vi "setUp.vi"(8 "error in (no error)":errorcluster, 11 "reference in":refnum<class "Switch Consumer Test Case.lvclass">) -> (0 "error out":errorcluster, 3 "reference out":refnum<class "Switch Consumer Test Case.lvclass">)   [LabVIEW 2017, in "Switch Consumer Test Case.lvclass"]
doc: "setUp runs prior to the test method during test execution. Use this method to initialize any object data required by your tests."
uses:
  Switch Consumer Test Case.lvclass
  C:/Program Files (x86)/National Instruments/LabVIEW 2017/vi.lib/addons/_JKI Toolkits/VI Tester/TestCase.llb/TestCase.lvclass
  Support/Switch/Test Switch Consumer/Test Switch Consumer.lvclass
  C:/github/niveristand-custom-device-message-library/Source/Consumer/Abstract Consumer/Abstract Consumer.lvclass
  Support/Switch/Test Switch Init Parameters/Test Switch Init Parameters.lvclass
  C:/github/niveristand-custom-device-message-library/Source/Parameters/Abstract Init Parameters/Abstract Init Parameters.lvclass
  C:/github/niveristand-custom-device-message-library/Source/Switch/Abstract Switch Init Parameters/Abstract Switch Init Parameters.lvclass
  Message Queue/Message Queue/Message Queue.lvclass
  C:/github/niveristand-custom-device-message-library/Source/Message Queue/Abstract Message Queue/Abstract Message Queue.lvclass
  Parameters/Abstract Init Parameters/Abstract Init Parameters.lvclass
  Producer/Abstract Producer/Abstract Producer.lvclass
  Support/Message String Action.ctl
  Support/Message List Action.ctl
  Support/Switch/Test Switch Init Parameters/Test Switch Init Parameters.lvclass/Test Switch Init Parameters.ctl
  Switch Consumer Test Case.lvclass/Switch Consumer Test Case.ctl
  Support/Switch/Test Switch Init Parameters/Write Test Param.vi
  <vilib>/addons/_JKI Toolkits/VI Tester/TestCase.llb/TestCase.lvclass
  Consumer/Abstract Consumer/Abstract Consumer.lvclass
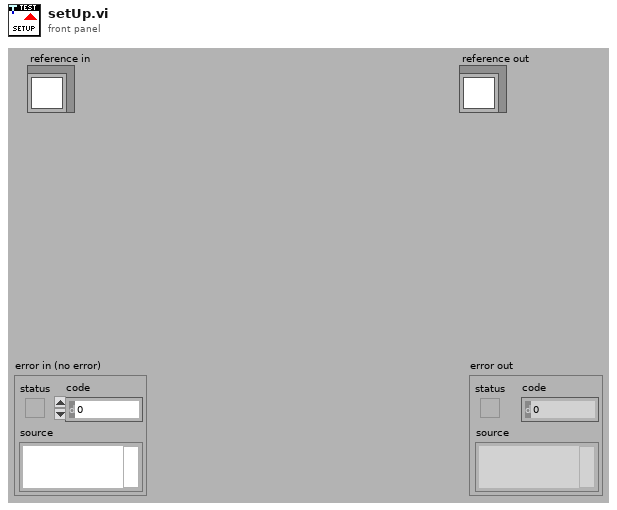
[diagram p1: front panel]
types:
  T1 = typedef "Message List Action.ctl" = enum16{"Get", "Add", "Reset"}
  T2 = typedef "Message String Action.ctl" = enum16{"Get String", "Set String", "Reset"}
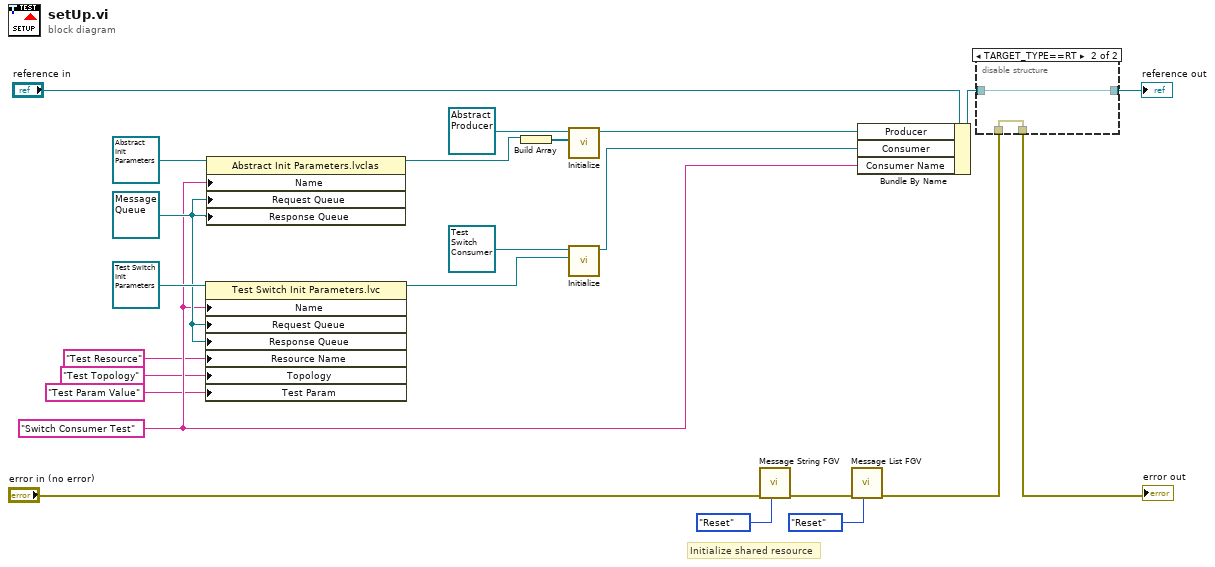
[diagram p0: block diagram]
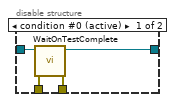
[diagram p2: hidden frame]
diagram:
  w9 = "Switch Consumer Test" ("Name")
  w17 = refnum<class "Message Queue.lvclass"> refnum ("Messaging.lvlib:Message Queue.lvlib:Message Queue.lvclass")
  # "Initialize shared resource"
  n1 = property class="Test Switch Init Parameters.lvc"(reference=refnum<class "Test Switch Init Parameters.lvclass"> refnum ("Test Switch Init Parameters.lvclass"), "Name"=w9, "Request Queue"=w17, "Response Queue"=w17, "Resource Name"="Test Resource", "Topology"="Test Topology", "Test Param"="Test Param Value" ("Topology")) -> (reference out=w11:refnum<class "Test Switch Init Parameters.lvclass">)  [unwired: 1 in, 1 out]
  n2 = property class="Abstract Init Parameters.lvclas"(reference=refnum<class "Abstract Init Parameters.lvclass"> refnum ("Message Queue Library.lvlib:Abstract Init Parameters.lvclass"), "Name"=w9, "Request Queue"=w17, "Response Queue"=w17) -> (reference out=w14:refnum<class "Abstract Init Parameters.lvclass">)  [unwired: 1 in, 1 out]
  n3 = Build Array(w14) -> (w15:refnum<class "Abstract Init Parameters.lvclass">[])
  n4 = call "Initialize.vi"("Parameters in"=w15, "Abstract Producer in"=refnum<class "Abstract Producer.lvclass"> refnum ("Messaging.lvlib:Producer.lvlib:Abstract Producer.lvclass")) -> ("Abstract Producer out"=w13:refnum<class "Abstract Producer.lvclass">)  [unwired: 8 in, 1 out]
  n5 = call "Initialize.vi"("Parameters in"=w11, "Abstract Consumer in"=refnum<class "Test Switch Consumer.lvclass"> refnum ("Test Switch Consumer.lvclass")) -> ("Abstract Consumer out"=w10:refnum<class "Test Switch Consumer.lvclass">)  [unwired: 8 in, 1 out]
  n6 = call "Message String FGV.vi"("Action"=Message_String_Action."Reset", "error in (no error)"="error in (no error)") -> ("error out"=w6:errorcluster)  [unwired: 8 in, 1 out]
  n7 = call "Message List FGV.vi"("Action (Get)"=Message_List_Action."Reset", "error in (no error)"=w6) -> ("error out"=w4:errorcluster)  [unwired: 8 in, 1 out]
  n8 = Bundle By Name(cluster="reference in", "Producer"=w13, "Consumer"=w10, "Consumer Name"=w9) -> (w20:refnum<class "Switch Consumer Test Case.lvclass">)
  n9 = disable-structure shown="TARGET_TYPE==RT" {
    disable-tunnel: w4 -> [w27 w28]
    disable-tunnel: [w26 w28] -> w23
    disable-tunnel: [w25 w29] -> w21
    disable-tunnel: w20 -> [w24 w29]
    frame condition #0 (active) {
      n10 = call <vilib>:"WaitOnTestComplete.vi"("error in (no error)"=w27, "TestCase in"=w24) -> ("error out"=w26:errorcluster, "TestCase out"=w25:refnum<class "Switch Consumer Test Case.lvclass">)  [unwired: 8 in]
    }
    frame condition #1 {
    }
  }
  "error out" <- w23
  "reference out" <- w21
